vi "Get Call Chain Prefix.vi"() -> (2 "Call Chain Prefix":string)   [LabVIEW 2013, in "JUnit for Azure Pipelines.lvclass"]
uses:
  JUnit for Azure Pipelines.lvclass
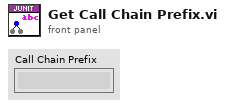
[diagram p1: front panel]
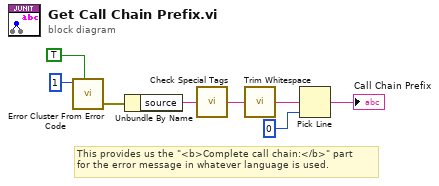
[diagram p0: block diagram]
diagram:
  # "This provides us the \"<b>Complete call chain:</b>\" part\nfor the error message in whatever language is used."
  n1 = call <vilib>:"Error Cluster From Error Code.vi"("show call chain? (False)"=TRUE, "error code (0)"=1) -> ("error out"=w6:errorcluster)  [unwired: 7 in]
  n2 = Unbundle By Name(w6) -> ("source"=w5:string)
  n3 = call <vilib>:"Check Special Tags.vi"("source"=w5) -> ("After Tag (special data)"=w4:string)  [unwired: 2 out]
  n4 = call <vilib>:"Trim Whitespace.vi"("string"=w4) -> ("trimmed string"=w3:string)  [unwired: 1 in]
  n5 = Pick Line(multi-line string=w3, line index=0) -> (output string=→"Call Chain Prefix":string)  [unwired: 1 in]
